vi "Rising Edge Detector.vi"(1 "Signal In":bool) -> (0 "Edge Detected?":bool)   [LabVIEW 2011]
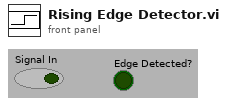
[diagram p1: front panel]
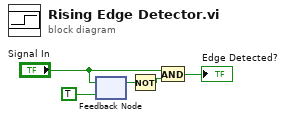
[diagram p0: block diagram]
diagram:
  n1 = feedback-in #1("Signal In") -> ()
  n2 = feedback #1(TRUE) -> (w4:bool)
  n3 = Not(x=w4) -> (.not. x?=w5:bool)
  n4 = And(x="Signal In", y=w5) -> (x .and. y?=→"Edge Detected?":bool)
